vi "LIA 2SOS.vi"(5 "lock-in.iir enable0 0":bool, 6 "lock-in.iir config0 0":T2, 7 "lock-in.iir decimation0 0":fxp<+,4,4>, 9 "input valid":bool, 11 "IQ_Data_In":T1) -> (1 "output valid":bool, 3 "IQ_Data_Out":T1)   [LabVIEW 2018]
uses:
  <instrlib>/_niInstr/DSP/v1/Shared/Public/IQ Data.ctl
  Shared/SOS/Controls/IIR_Coeffs.ctl
  <instrlib>/_niInstr/DSP/v1/Shared/niInstr DSP v1 Shared.lvlib
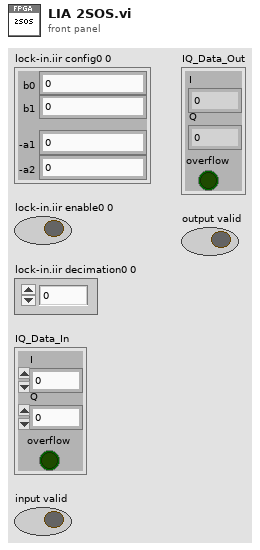
[diagram p1: front panel]
types:
  T1 = typedef "niInstr DSP v1 Shared.lvlib/IQ Data.ctl" = cluster{"I":fxp<+/-,18,1>, "Q":fxp<+/-,18,1>, "overflow":bool}
  T2 = typedef "IIR_Coeffs.ctl" = cluster{"b0":fxp<+/-,18,2>, "b1":fxp<+/-,18,2>, "-a1":fxp<+/-,18,2>, "-a2":fxp<+/-,18,2>}
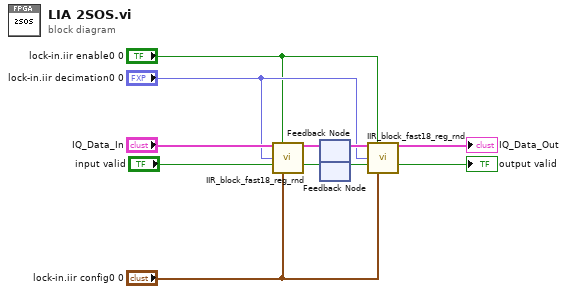
[diagram p0: block diagram]
diagram:
  n1 = call "IIR_block_fast18_reg_rnd.vi"("IQ_Data_In"="IQ_Data_In", "enable"="lock-in.iir enable0 0", "Decimation Factor (-1)"="lock-in.iir decimation0 0", "Valid In"="input valid", "IIR 2 coeffs"="lock-in.iir config0 0") -> ("IQ_Data_Out"=w1:T1, "output valid"=w3:bool)  [unwired: 9 in]
  n2 = feedback #1() -> (w10:T1)  [unwired: 1 in]
  n3 = feedback-in #1(w1) -> ()
  n4 = feedback #2() -> (w11:bool)  [unwired: 1 in]
  n5 = feedback-in #2(w3) -> ()
  n6 = call "IIR_block_fast18_reg_rnd.vi"("IQ_Data_In"=w10, "enable"="lock-in.iir enable0 0", "Decimation Factor (-1)"="lock-in.iir decimation0 0", "Valid In"=w11, "IIR 2 coeffs"="lock-in.iir config0 0") -> ("IQ_Data_Out"=→"IQ_Data_Out":T1, "output valid"=→"output valid":bool)  [unwired: 9 in]
